vi "IMAQController.ProcCases.vi"(0 "i ref in":refnum<vi>, 1 "selector":string, 2 "Data":T3, 3 "call cluster":T1={"Object"="", "Selector"="", "CallType"=enum."synchronous", "Async Object"="", "Async Selector"="", "Data Descriptor"="", "Data"=[], "Error #"=0, "Expire"=0}, 5 "error in (no error)":errorcluster) -> (14 "i ref out":refnum<vi>, 17 "answer cluster":T1={"Object"="", "Selector"="", "CallType"=enum."synchronous", "Async Object"="", "Async Selector"="", "Data Descriptor"="", "Data"=[], "Error #"=0, "Expire"=0}, 19 "error out":errorcluster)   [LabVIEW 2014, in "IMAQController.lvlib"]
uses:
  IMAQController.lvlib
  CSCore/CSSystem/CoreDefs/CoreDefs.rawDataType.ctl
  CSCore/CSSystem/CoreDefs/CoreDefs.call_type.ctl
  CSCore/BaseProcess/BaseProcess.descriptor string definition.ctl
  CSCore/BaseProcess/BaseProcess.lvlib
  CSCore/CSObj/CSObj.lvlib
  CSlibraries-extern/DimLVEvent/LVDimInterface/LVDimInterface.lvlib
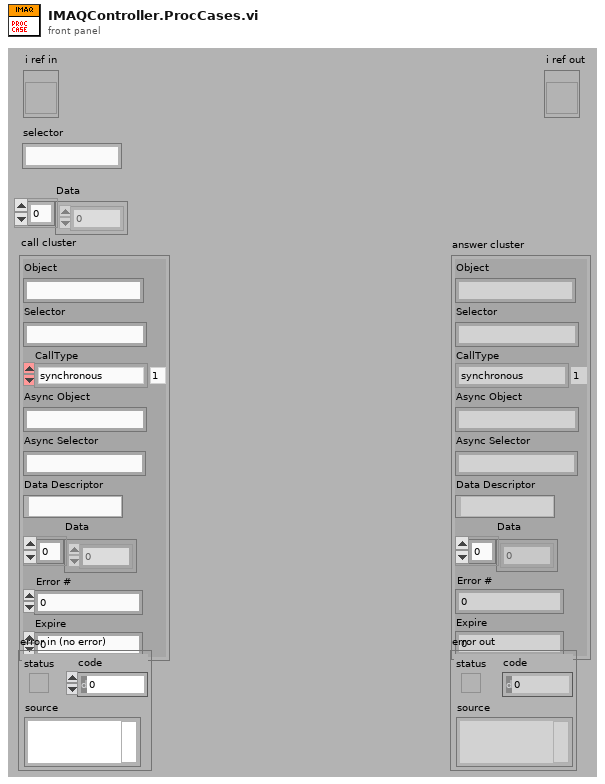
[diagram p1: front panel]
types:
  T1 = typedef "CoreDefs.call_type.ctl" = cluster{"Object":string, "Selector":string, "CallType":enum16{"simple", "synchronous", "asynchronous"}, "Async Object":string, "Async Selector":string, "Data Descriptor":T2, "Data":T3, "Error #":i32, "Expire":u32}
  T2 = typedef "BaseProcess.lvlib/BaseProcess.descriptor string definition.ctl" = string
  T3 = typedef "CoreDefs.rawDataType.ctl" = i8[]
  T4 = typedef "IMAQController.lvlib/IMAQController.i attribute.ctl" = cluster{"ImageTakenID":i32, "actSequencer":string, "actScanner":string, "CameraTriggerID":i32, "activatedCameras":cluster{"Name":string, "Camera Type":string, "Acquisition Mode":u32, "JPEG Mode?":bool, "Acquisition Delay":dbl, "Save Images?":bool, "Center Coordinates":T5, "PixelPermm":cluster{"Horizontal":dbl, "Vertical":dbl}, "Rotation":dbl, "Mirror Mode":u32, "PixelCoordinates":cluster{"1":cluster{"Horizontal":i32, "Vertical":i32}, "2":cluster{"Horizontal":i32, "Vertical":i32}, "3":cluster{"Horizontal":i32, "Vertical":i32}, "4":cluster{"Horizontal":i32, "Vertical":i32}}, "RWCoordinates":cluster{"1":cluster{"Horizontal":dbl, "Vertical":dbl}, "2":cluster{"Horizontal":dbl, "Vertical":dbl}, "3":cluster{"Horizontal":dbl, "Vertical":dbl}, "4":cluster{"Horizontal":dbl, "Vertical":dbl}}, "HorizScaling":dbl, "VertScaling":dbl}[], "Ini C-Array":string[], "actCamera":string, "activeCamera":cluster{"Name":string, "Camera Type":string, "Aqcuisation Mode":enum32{"Internal Trigger", "Scan", "free Running", "External Trigger"}, "JPEG Mode?":bool, "Acquisition Delay":dbl, "Save Images?":bool, "Center Coordinates":T5, "PixelPermm":cluster{"Horizontal":dbl, "Vertical":dbl}, "Rotation":dbl, "Mirror Mode":u32, "PixelCoordinates":cluster{"1":cluster{"Horizontal":i32, "Vertical":i32}, "2":cluster{"Horizontal":i32, "Vertical":i32}, "3":cluster{"Horizontal":i32, "Vertical":i32}, "4":cluster{"Horizontal":i32, "Vertical":i32}}, "RWCoordinates":cluster{"1":cluster{"Horizontal":dbl, "Vertical":dbl}, "2":cluster{"Horizontal":dbl, "Vertical":dbl}, "3":cluster{"Horizontal":dbl, "Vertical":dbl}, "4":cluster{"Horizontal":dbl, "Vertical":dbl}}, "HorizScaling":dbl, "VertScaling":dbl}, "BilderMittelungen":u8, "OldPicture":dbl[][]}
  T5 = typedef "LVPoint32TypeDef.ctl" = cluster{"Horizontal":i32, "Vertical":i32}
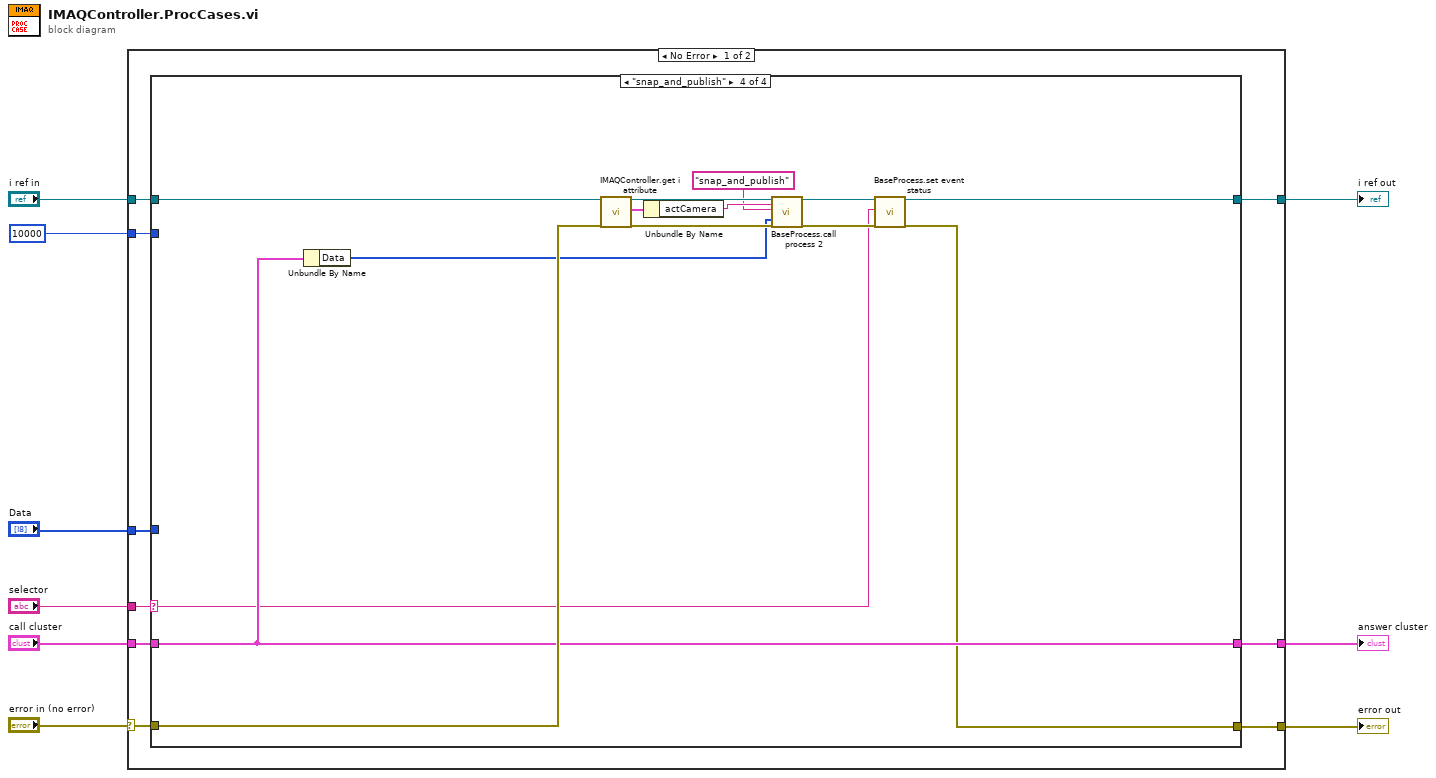
[diagram p0: block diagram]
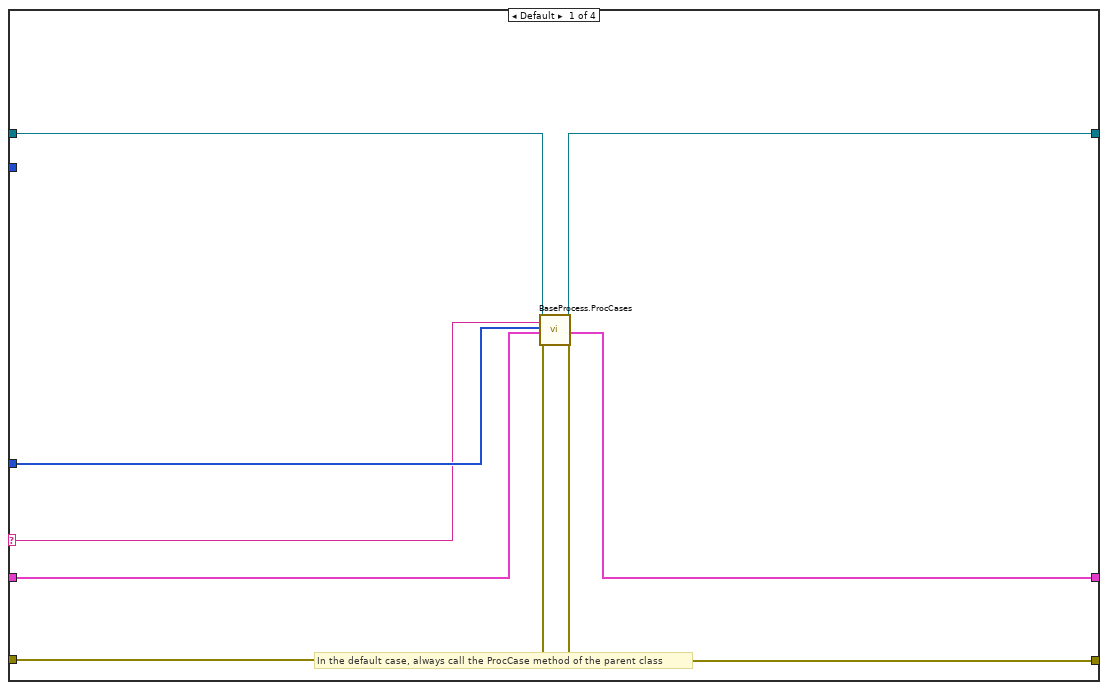
[diagram p2: hidden frame]
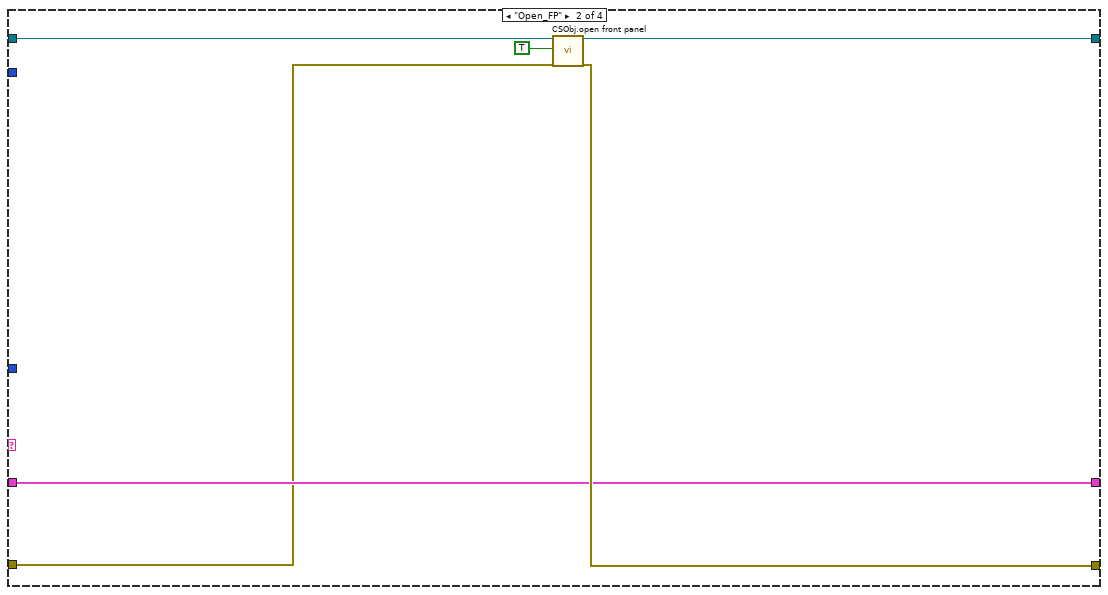
[diagram p3: hidden frame]
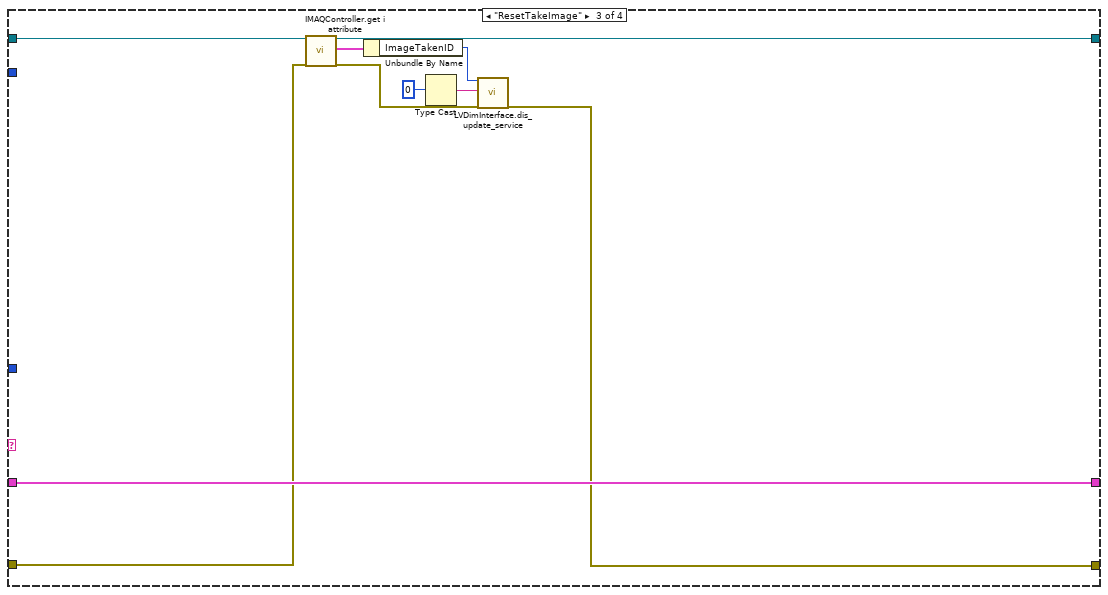
[diagram p4: hidden frame]
diagram:
  n1 = case shown="No Error" "error in (no error)" {
    selector: "error in (no error)" -> [w10 w57]
    tunnel: "selector" -> [w18 _]
    tunnel: [w17 w58] -> w8
    tunnel: "Data" -> [w16 _]
    tunnel: "call cluster" -> [w15 w58]
    tunnel: "i ref in" -> [w14 w59]
    tunnel: [w13 w59] -> w4
    tunnel: [w12 w57] -> w3
    tunnel: 10000 -> [w11 _]
    frame No Error {
      n2 = case shown="\"snap_and_publish\"" w18 {
        selector: w18 -> [w20 _ _ w43]
        tunnel: w16 -> [w21 _ _ _]
        tunnel: w14 -> [w19 w29 w41 w56]
        tunnel: [w26 w28 w40 w46] -> w13
        tunnel: w15 -> [w22 w30 w42 w54]
        tunnel: [w23 w30 w42 w54] -> w17
        tunnel: w10 -> [w25 w27 w39 w55]
        tunnel: [w24 w31 w37 w44] -> w12
        tunnel: w11 -> [_ _ _ _]
        frame Default {
          # "In the default case, always call the ProcCase method of the parent class"
          n3 = call "BaseProcess.ProcCases.vi"("i ref in"=w19, "selector"=w20, "Data"=w21, "call cluster"=w22, "error in (no error)"=w25) -> ("i ref out"=w26:refnum<vi>, "answer cluster"=w23:T1, "error out"=w24:errorcluster)  [unwired: 12 in]
        }
        frame "Open_FP" {
          n4 = call "CSObj.open front panel.vi"("i ref in"=w29, "frontPanelOpen"=TRUE ("front panel open"), "error in (no error)"=w27) -> ("i ref out"=w28:refnum<vi>, "error out"=w31:errorcluster)  [unwired: 15 in]
        }
        frame "ResetTakeImage" {
          n5 = call "IMAQController.get i attribute.vi"("i ref in"=w41, "error in (no error)"=w39) -> ("i ref out"=w40:refnum<vi>, "i attribute"=w34:T4, "error out"=w38:errorcluster)  [unwired: 15 in]
          n6 = Unbundle By Name(w34) -> ("ImageTakenID"=w33:i32)
          n7 = Type Cast(x=i16 0) -> (*(type *) &x=w35:string)  [unwired: 1 in]
          n8 = call "LVDimInterface.dis_update_service.vi"("my_serviceID"=w33, "data"=w35, "error in (no error)"=w38) -> ("error out"=w37:errorcluster)  [unwired: 14 in, 2 out]
        }
        frame "snap_and_publish" {
          n9 = Unbundle By Name(w54) -> ("Data"=w48:T3)
          n10 = call "IMAQController.get i attribute.vi"("i ref in"=w56, "error in (no error)"=w55) -> ("i ref out"=w52:refnum<vi>, "i attribute"=w53:T4, "error out"=w49:errorcluster)  [unwired: 15 in]
          n11 = Unbundle By Name(w53) -> ("actCamera"=w51:string)
          n12 = call "BaseProcess.call process 2.vi"("i ref in"=w52, "Object"=w51, "Selector"="snap_and_publish", "Data"=w48, "error in (no error)"=w49) -> ("i ref out"=w47:refnum<vi>, "error out"=w45:errorcluster)  [unwired: 13 in]
          n13 = call "BaseProcess.set event status.vi"("i ref in"=w47, "EventStatus"=w43, "error in (no error)"=w45) -> ("i ref out"=w46:refnum<vi>, "error out"=w44:errorcluster)  [unwired: 14 in, 1 out]
        }
      }
    }
    frame Error {
    }
  }
  "answer cluster" <- w8
  "i ref out" <- w4
  "error out" <- w3
